vi "Calculate Acquisition Length - Sine.vi"(9 "number of cycles to acquire":u32, 10 "input frequency":dbl, 11 "sample rate":u32) -> (1 "actual number of cycles":u32, 2 "acquisition duration":dbl, 3 "samples to acquire":u32)   [LabVIEW 2021]
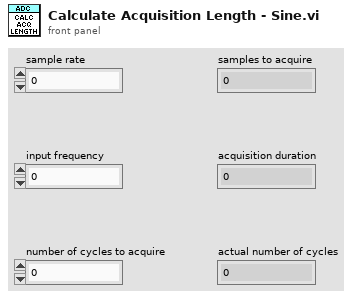
[diagram p1: front panel]
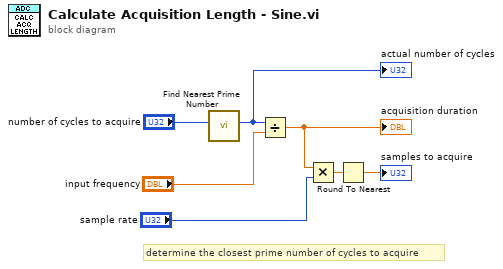
[diagram p0: block diagram]
diagram:
  # "determine the closest prime number of cycles to acquire"
  n1 = call "Find Nearest Prime Number.vi"("start number"="number of cycles to acquire") -> ("prime number"=w6:u32)  [unwired: 10 in]
  "actual number of cycles" <- w6
  n2 = Divide(x=w6, y="input frequency") -> (x/y=w4:dbl)
  "acquisition duration" <- w4
  n3 = Multiply(x=w4, y="sample rate") -> (x*y=w2:dbl)
  n4 = Round To Nearest(number=w2) -> (nearest integer value=→"samples to acquire":dbl)
